vi "PM100D_GetSystemInfo.vi"(0 "VISA in":refnum<visa-resource-name>, 1 "error in":errorcluster) -> (2 "VISA out":refnum<visa-resource-name>, 3 "Instrument":string, 4 "SN":string, 5 "error out":errorcluster)   [LabVIEW 2010]
doc: "Get device name and serial number"
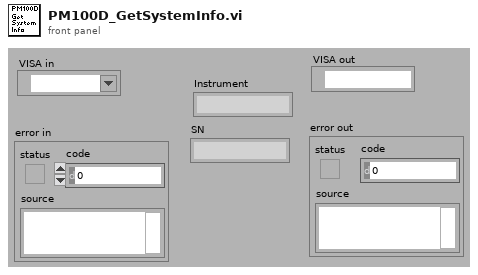
[diagram p1: front panel]
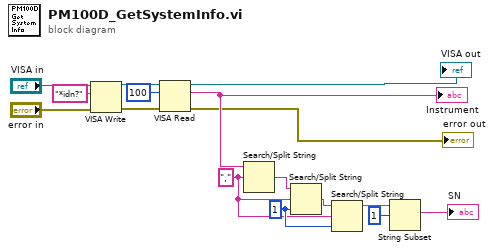
[diagram p0: block diagram]
diagram:
  w13 = 1 ("offset (0)")
  w12 = "," ("search string/char (-)")
  n1 = VISA Write(VISA resource name="VISA in", write buffer="*idn?", error in (no error)="error in") -> (VISA resource name out=w3:refnum<visa-resource-name>, error out=w6:errorcluster)  [unwired: 1 out]
  n2 = VISA Read(VISA resource name=w3, byte count=u32 100, error in (no error)=w6) -> (VISA resource name out=→"VISA out":refnum<visa-resource-name>, read buffer=w8:string, error out=→"error out":errorcluster)  [unwired: 1 out]
  "Instrument" <- w8
  n3 = Search/Split String(string=w8, search string/char (-)=w12) -> (match + rest of string=w10:string)  [unwired: 3 out]
  n4 = Search/Split String(string=w10, search string/char (-)=w12, offset (0)=w13) -> (match + rest of string=w11:string)  [unwired: 2 out]
  n5 = Search/Split String(string=w11, search string/char (-)=w12, offset (0)=w13) -> (substring before match=w14:string)  [unwired: 2 out]
  n6 = String Subset(string=w14, offset (0)=1) -> (substring=→"SN":string)  [unwired: 1 out]
